vi "MAIN_change_illumination.vi"(5 "Illumination Refnum":refnum<vi>, 6 "task number":i32, 8 "error in":errorcluster, 9 "Illumination control":T1 {"641" min=0.0 max=100.0 step=0.10000000149011612 scale=0.0..100.0; "561" min=0.0 max=100.0 step=0.10000000149011612 scale=0.0..100.0; "405" min=0.0 max=100.0 step=0.10000000149011612 scale=0.0..100.0; "488" min=0.0 max=100.0 step=0.10000000149011612 scale=0.0..100.0; "BF" min=0.0 max=100.0 step=0.1 scale=0.0..100.0}, 10 "queue ASI stage":refnum<queue>, 11 "queue FPGA":refnum<queue>) -> (0 "error out":errorcluster)   [LabVIEW 2015]
uses:
  CONTROLS/Q_ASI_stage_element.ctl
  CONTROLS/Illumination and filters.ctl
  CONTROLS/Q_FPGA_element.ctl
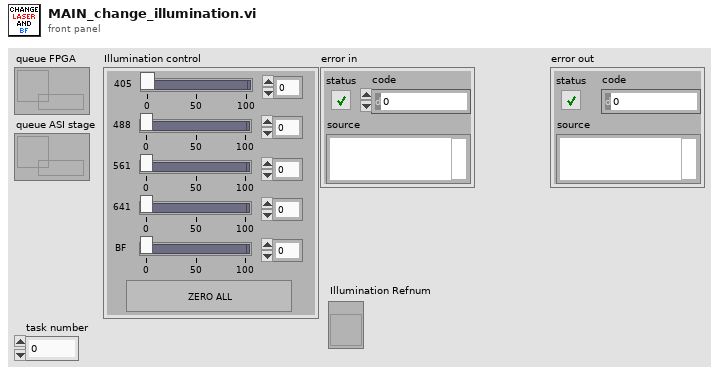
[diagram p1: front panel]
types:
  T1 = typedef "Illumination and filters.ctl" = cluster{"BF ":dbl, "641":dbl, "561":dbl, "488":dbl, "405":dbl, "ZERO ALL":bool}
  T2 = typedef "Q_ASI_stage_element.ctl" = cluster{"variant":variant, "Instruction":enum16{"ASI_idle", "ASI_initialize", "ASI_error", "ASI_security_stop", "ASI_read_XYZ", "ASI_up", "ASI_down", "ASI_left", "ASI_right", "ASI_save_XY", "ASI_move_to_XY", "ASI_brightfield", "ASI_init_scan", "ASI_init_merFISH", "ASI_move_to_XY_merFISH", "ASI_move_to_Z_merFISH", "ASI_init_autofocus_search_merFISH", "ASI_close_autofocus_search_merFISH", "ASI_adjust_piezo_autofocus_merFISH", "ASI_set_piezo_autofocus_to_reference_position_merFISH_TL", "ASI_close_merFISH", "ASI_stop"}}
  T3 = typedef "Q_FPGA_element.ctl" = cluster{"variant":variant, "Instruction":enum16{"FPGA_idle", "FPGA_initialize", "FPGA_error", "FPGA_security_stop", "FPGA_laser", "FPGA_start_stop_measure_QPD", "FPGA_measure_QPD", "FPGA_measure_QPD_noise", "FPGA_stop_measure_QPD", "FPGA_init_autofocus", "FPGA_init_single_scan", "FPGA_stop_single_scan", "FPGA_init_merFISH", "FPGA_measure_QPD_merFISH", "FPGA_init_scan_merFISH", "FPGA_scan_merFISH", "FPGA_close_merFISH", "FPGA_stop"}}
  T4 = cluster{"561":sgl, "641":sgl, "405":sgl, "488":sgl}
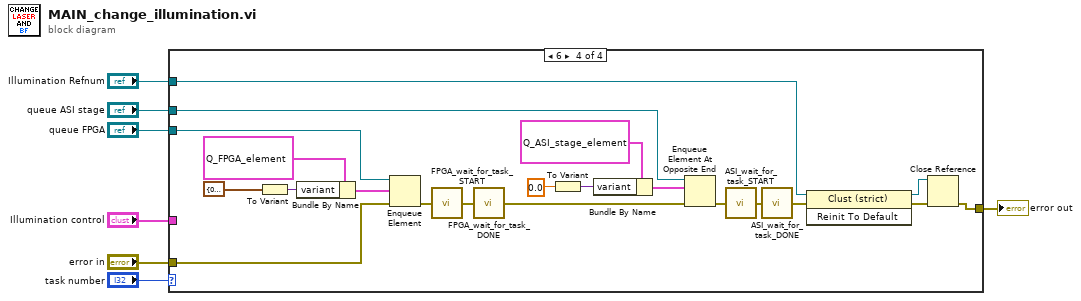
[diagram p0: block diagram]
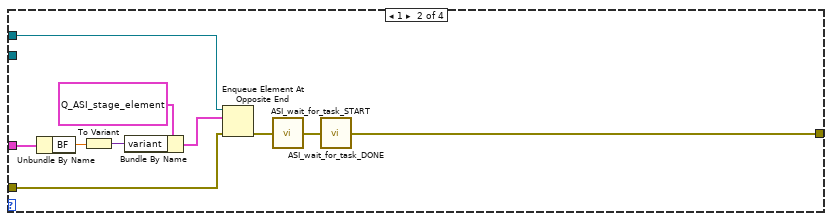
[diagram p3: hidden frame]
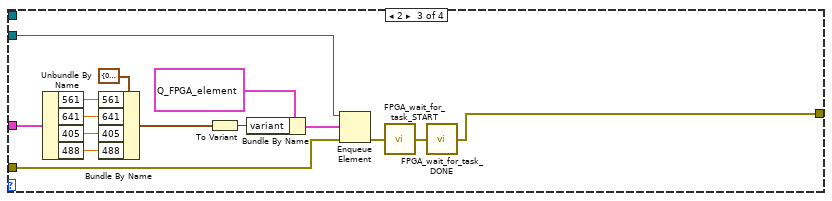
[diagram p4: hidden frame]
diagram:
  n1 = case shown="6" "task number" {
    tunnel: "Illumination control" -> [_ w17 w33 _]
    tunnel: "error in" -> [w8 w15 w26 w38]
    tunnel: "queue FPGA" -> [_ _ w27 w37]
    tunnel: [w8 w9 w19 w53] -> w3
    tunnel: "queue ASI stage" -> [_ w12 _ w43]
    tunnel: "Illumination Refnum" -> [_ _ _ w51]
    frame 0, Default {
    }
    frame 1 {
      n2 = Unbundle By Name(w17) -> ("BF"=w13:dbl)
      n3 = To Variant(anything=w13) -> (Variant=w18:variant)
      n4 = Bundle By Name(cluster=T2 {"variant"=variant, "Instruction"=enum."ASI_brightfield"} ("Q_ASI_stage"), "variant"=w18) -> (w16:T2)
      n5 = Enqueue Element At Opposite End(queue=w12, element=w16, error in (no error)=w15) -> (error out=w14:errorcluster)  [unwired: 1 in, 2 out]
      n6 = call "ASI_wait_for_task_START.vi"("error in"=w14) -> ("error out"=w10:errorcluster)
      n7 = call "ASI_wait_for_task_DONE.vi"("error in"=w10) -> ("error out"=w9:errorcluster)
    }
    frame 2 {
      n8 = Unbundle By Name(w33) -> ("561"=w31:dbl, "641"=w30:dbl, "405"=w29:dbl, "488"=w28:dbl)
      n9 = Bundle By Name(cluster=T4 {"561"=0.0, "641"=0.0, "405"=0.0, "488"=0.0} ("output cluster"), "561"=w31, "641"=w30, "405"=w29, "488"=w28) -> (w23:T4)
      n10 = To Variant(anything=w23) -> (Variant=w24:variant)
      n11 = Bundle By Name(cluster=T3 {"variant"=variant, "Instruction"=enum."FPGA_laser"} ("element"), "variant"=w24) -> (w22:T3)
      n12 = Enqueue Element(queue=w27, element=w22, error in (no error)=w26) -> (error out=w21:errorcluster)  [unwired: 1 in, 2 out]
      n13 = call "FPGA_wait_for_task_START.vi"("error in"=w21) -> ("error out"=w20:errorcluster)
      n14 = call "FPGA_wait_for_task_DONE.vi"("error in"=w20) -> ("error out"=w19:errorcluster)
    }
    frame 6 {
      n15 = To Variant(anything=T4 {"561"=0.0, "641"=0.0, "405"=0.0, "488"=0.0} ("output cluster")) -> (Variant=w41:variant)
      n16 = Bundle By Name(cluster=T3 {"variant"=variant, "Instruction"=enum."FPGA_laser"} ("element"), "variant"=w41) -> (w40:T3)
      n17 = Enqueue Element(queue=w37, element=w40, error in (no error)=w38) -> (error out=w39:errorcluster)  [unwired: 1 in, 2 out]
      n18 = call "FPGA_wait_for_task_START.vi"("error in"=w39) -> ("error out"=w35:errorcluster)
      n19 = call "FPGA_wait_for_task_DONE.vi"("error in"=w35) -> ("error out"=w34:errorcluster)
      n20 = To Variant(anything=0.0 ("BF")) -> (Variant=w49:variant)
      n21 = Bundle By Name(cluster=T2 {"variant"=variant, "Instruction"=enum."ASI_brightfield"} ("Q_ASI_stage"), "variant"=w49) -> (w48:T2)
      n22 = Enqueue Element At Opposite End(queue=w43, element=w48, error in (no error)=w34) -> (error out=w44:errorcluster)  [unwired: 1 in, 2 out]
      n23 = call "ASI_wait_for_task_START.vi"("error in"=w44) -> ("error out"=w50:errorcluster)
      n24 = call "ASI_wait_for_task_DONE.vi"("error in"=w50) -> ("error out"=w45:errorcluster)
      n25 = invoke class="Clust (strict)" method="Reinit To Default"(reference=w51, error in=w45) -> (reference out=w52:refnum<vi>, error out=w54:errorcluster)  [unwired: 1 in, 1 out]
      n26 = Close Reference(reference=w52, error in (no error)=w54) -> (error out=w53:errorcluster)
    }
  }
  "error out" <- w3
